vi "PAS Core.vi"(10 "nPAS In":refnum<class "nPAS.lvclass">, 11 "DVR In":refnum<data-value>) -> (3 "nPAS out":refnum<class "nPAS.lvclass">)   [LabVIEW 2015]
uses:
  Data/Nicholas Data.lvclass
  PAS/nPAS.lvclass
  Reusable/Instrument/state.ctl
  Reusable/Session Log/System Log.lvclass
  Reusable/Session APIs/File Access/Config Data/Config Data.lvclass
  Reusable/Session Log/System Log.lvclass/System Log.ctl
  Reusable/Session APIs/File Access/Config Data/Config Data.lvclass/Config Data.ctl
  Reusable/Instrument/Instrument.lvclass/Instrument.ctl
  PAS/nPAS.lvclass/nPAS.ctl
  Reusable/Session Log/Accessors/Write Main Path.vi
  Reusable/Session APIs/File Access/Config Data/Accessors/Write Cfg Path.vi
  Reusable/Instrument/Write Log Session.vi
  Reusable/Instrument/Write Cfg Session.vi
  Reusable/Instrument/Instrument.lvclass
  <userlib>/_Session Fwk/Session - Root.lvclass
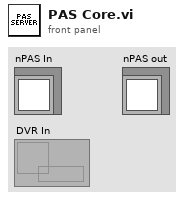
[diagram p1: front panel]
types:
  T1 = typedef "Instrument.lvclass/state.ctl" = enum8{"Configure", "Acquire", "Wait", "Quit", "Handle Error", "NOOP"}
  T2 = typedef "Session - Root.lvclass/Session Handle.ctl" = refnum<data-value>
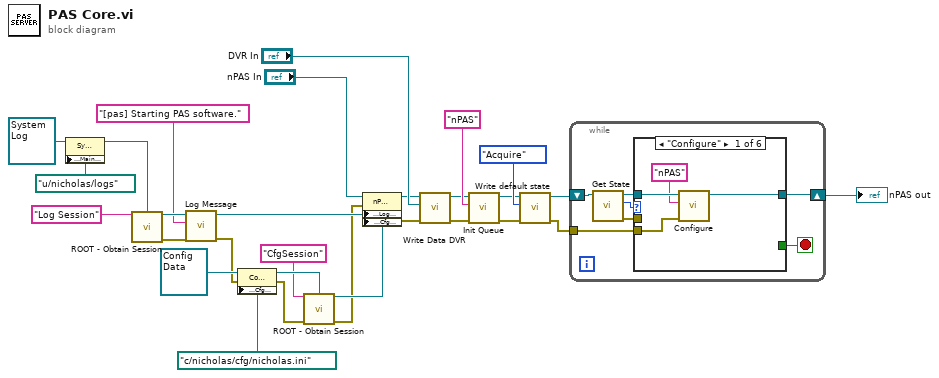
[diagram p0: block diagram]
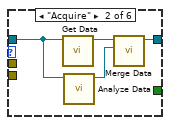
[diagram p2: hidden frame]
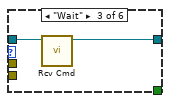
[diagram p3: hidden frame]
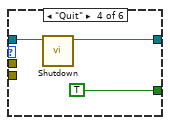
[diagram p4: hidden frame]
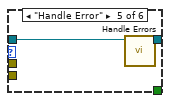
[diagram p5: hidden frame]
diagram:
  n1 = property class="Sys Log"(reference=refnum<class "System Log.lvclass"> refnum ("Sys Log"), "Accessors:Main Path"=path "u:/nicholas/logs" ("Main Path")) -> (reference out=w17:refnum<class "System Log.lvclass">)  [unwired: 1 in, 1 out]
  n2 = call <userlib>:"ROOT - Obtain Session.vi"("Session Name ()"="Log Session", "OBJ - Session"=w17) -> ("Session Handle"=w15:T2, "error out"=w10:errorcluster)  [unwired: 11 in, 1 out]
  n3 = call "Log Message.vi"("error in"=w10, "MSG In"="[pas] Starting PAS software.", "session in"=w15) -> ("error out"=w3:errorcluster, "session out"=w11:T2)  [unwired: 7 in]
  n4 = property class="Config Data"(reference=refnum<class "Config Data.lvclass"> refnum ("Config Data"), error in=w3, "Accessors:Cfg Path"=path "c:/nicholas/cfg/nicholas.ini" ("Cfg Path")) -> (reference out=w7:refnum<class "Config Data.lvclass">, error out=w2:errorcluster)
  n5 = call <userlib>:"ROOT - Obtain Session.vi"("Session Name ()"="CfgSession", "OBJ - Session"=w7, "error in (no error)"=w2) -> ("Session Handle"=w5:T2, "error out"=w4:errorcluster)  [unwired: 10 in, 1 out]
  n6 = property class="nPAS"(reference="nPAS In", error in=w4, "Accessors:Log Session"=w11, "Accessors:Cfg Session"=w5) -> (reference out=w12:refnum<class "nPAS.lvclass">, error out=w1:errorcluster)
  n7 = call "Write Data DVR.vi"("error in (no error)"=w1, "Data DVR"="DVR In", "nPAS in"=w12) -> ("error out"=w20:errorcluster, "nPAS out"=w23:refnum<class "nPAS.lvclass">)  [unwired: 7 in]
  n8 = call "Init Queue.vi"("error in"=w20, "queue_name"="nPAS", "Instrument in"=w23) -> ("error out"=w25:errorcluster, "Instrument out"=w26:refnum<class "nPAS.lvclass">)  [unwired: 7 in]
  n9 = call "Write default state.vi"("error in (no error)"=w25, "instr state"=state."Acquire", "Instrument in"=w26) -> ("error out"=w29:errorcluster, "Instrument out"=w28:refnum<class "nPAS.lvclass">)  [unwired: 7 in]
  n10 = while {
    shift-right: [w34] -> w21
    shift-left: w28 -> [w35]
    tunnel: w29 -> [w33]
    stop <- w36 stop-if-true
    n11 = call "Get State.vi"("Instrument in"=w35) -> ("error out"=w30:errorcluster, "default state"=w32:T1, "Instrument out"=w31:refnum<class "nPAS.lvclass">)  [unwired: 8 in]
    n12 = case shown="\"Configure\"" w32 {
      tunnel: [_ _ _ TRUE _ _] -> w36
      tunnel: w31 -> [w40 w44 w46 w48 w51 w52]
      tunnel: [w39 w43 w45 w47 w50 w52] -> w34
      tunnel: w33 -> [w38 _ _ _ _ _]
      tunnel: w30 -> [_ _ _ _ _ _]
      frame "Configure" {
        n13 = call-dynamic "Configure.vi"("error in"=w38, "name"="nPAS", "nPAS in"=w40) -> ("nPAS out"=w39:refnum<class "nPAS.lvclass">)  [unwired: 7 in, 1 out]
      }
      frame "Acquire" {
        n14 = call-dynamic "Get Data.vi"("nPAS in"=w44) -> ("nPAS out"=w42:refnum<class "nPAS.lvclass">)  [unwired: 9 in, 1 out]
        n15 = call-dynamic "Analyze Data.vi"("nPAS in"=w44) -> ("nPAS out"=w41:refnum<class "nPAS.lvclass">)  [unwired: 9 in, 1 out]
        n16 = call-dynamic "Merge Data.vi"("Analyzed"=w41, "Acquired"=w42) -> ("PAS out"=w43:refnum<class "nPAS.lvclass">)  [unwired: 8 in, 1 out]
      }
      frame "Wait" {
        n17 = call-dynamic "Rcv Cmd.vi"("nPAS in"=w46) -> ("nPAS out"=w45:refnum<class "nPAS.lvclass">)  [unwired: 9 in, 1 out]
      }
      frame "Quit" {
        n18 = call-dynamic "Shutdown.vi"("nPAS in"=w48) -> ("nPAS out"=w47:refnum<class "nPAS.lvclass">)  [unwired: 9 in, 1 out]
      }
      frame "Handle Error" {
        n19 = call-dynamic "Handle Errors.vi"("Instrument in"=w51) -> ("Instrument out"=w50:refnum<class "nPAS.lvclass">)  [unwired: 8 in, 2 out]
      }
      frame "NOOP", Default {
      }
    }
  }
  "nPAS out" <- w21
